vi "Water_tank_level_indicator.vi"() -> ()   [LabVIEW 2020]
panel:
  out "TANK EMPTY":bool
  out "HALF FULL\n  (50 Litre)":bool
  out "TANK FULL":bool
  in  "Stop":bool
  in  "Flow out ltr/s":dbl(slide) scale=0.0..10.0
  in  "Flow in ltr/s":dbl(slide) scale=0.0..10.0
  out "Water Tank":dbl(slide) scale=0.0..100.0
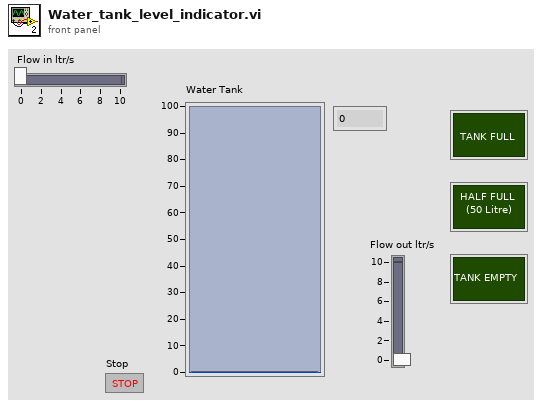
[diagram p1: front panel]
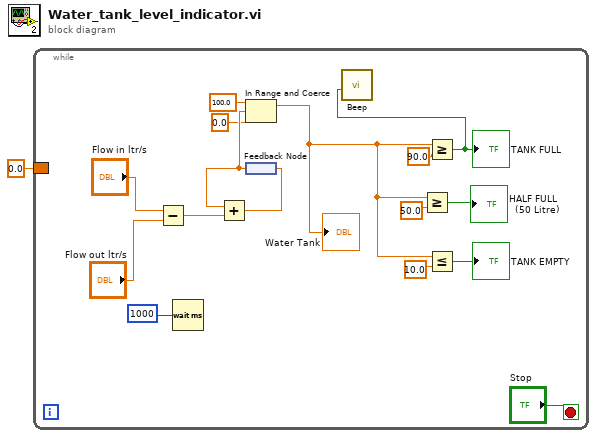
[diagram p0: block diagram]
diagram:
  n1 = while {
    border: 0.0 -> [_]
    stop <- "Stop" stop-if-true
    n2 = Subtract(x="Flow in ltr/s", y="Flow out ltr/s") -> (x-y=w14:dbl)
    n3 = Wait (ms)(milliseconds to wait=u32 1000 ("millisecond timer value")) -> ()  [unwired: 1 out]
    n4 = feedback #1() -> (w12:dbl)
    n5 = Add(x=w12, y=w14) -> (x+y=w13:dbl)
    n6 = In Range and Coerce(upper limit=100.0, x=w12, lower limit=0.0) -> (coerced(x)=w8:dbl)  [unwired: 1 out]
    "Water Tank" <- w8
    n7 = feedback-in #1(w13) -> ()
    n8 = Greater Or Equal?(x=w8, y=50.0) -> (x >= y?=→"HALF FULL\n  (50 Litre)":bool)
    n9 = Greater Or Equal?(x=w8, y=90.0) -> (x >= y?=w3:bool)
    "TANK FULL" <- w3
    n10 = call <vilib>:"Beep.vi"("use system alert? (T)"=w3) -> ()  [unwired: 11 in]
    n11 = Less Or Equal?(x=w8, y=10.0) -> (x <= y?=→"TANK EMPTY":bool)
  }
